vi "Print_a_spot.vi"(1 "Position":T1, 2 "String In":string) -> (0 "String Out":string)   [LabVIEW 2011]
doc: "for a position/location create a text line with comma delimited posiiton and name of postion. Formatted string includes: Name, X, Y, Z and a carriage return."
uses:
  cm2nm_coordinate_information_v2.ctl
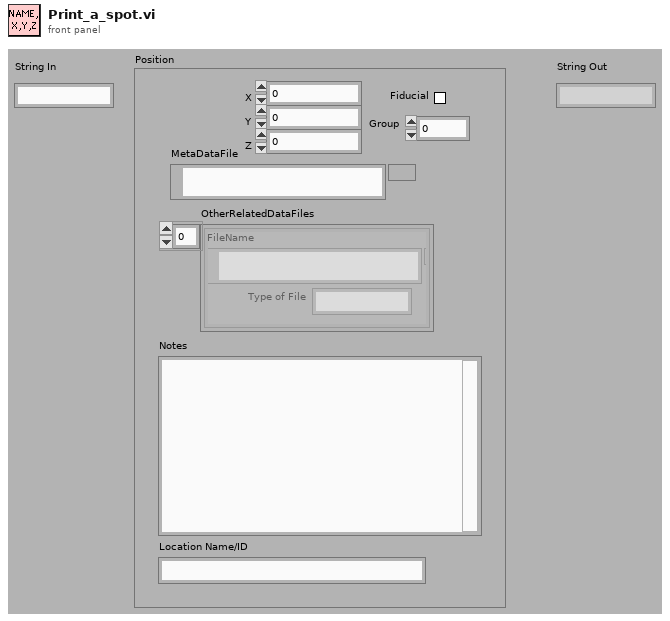
[diagram p1: front panel]
types:
  T1 = typedef "cm2nm_coordinate_information_v2.ctl" = cluster{"MetaDataFile":path, "X":dbl, "Y":dbl, "Z":dbl, "Group":i32, "Rotation":dbl[unit], "Fiducial":bool, "Magnification":dbl, "Working_Distance":dbl, "Notes":string, "Location Name/ID":string, "OtherRelatedDataFiles":cluster{"Type of File":string, "FileName":path}[], "Available":bool}
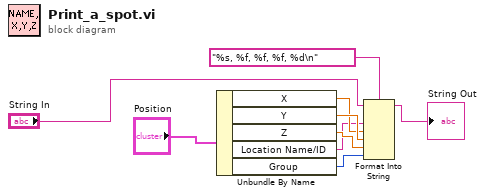
[diagram p0: block diagram]
diagram:
  n1 = Unbundle By Name("Position") -> ("X"=w6:dbl, "Y"=w7:dbl, "Z"=w8:dbl, "Location Name/ID"=w5:string, "Group"=w1:i32)
  n2 = Format Into String(format string="%s, %f, %f, %f, %d\n", initial string="String In", w5, w6, w7, w8, w1) -> (resulting string=→"String Out":string)  [unwired: 1 in, 1 out]
